vi "wait4.vi"(8 "error In":errorcluster, 9 "JSON string":string, 10 "Step order":string, 11 "process_ID":string) -> (0 "error IO":errorcluster)   [LabVIEW 2020]
uses:
  status/status of power_supply4.vi
  status/emergency stop.vi
  status/pause4.vi
  status/time4.vi
panel:
  out "current time":timestamp
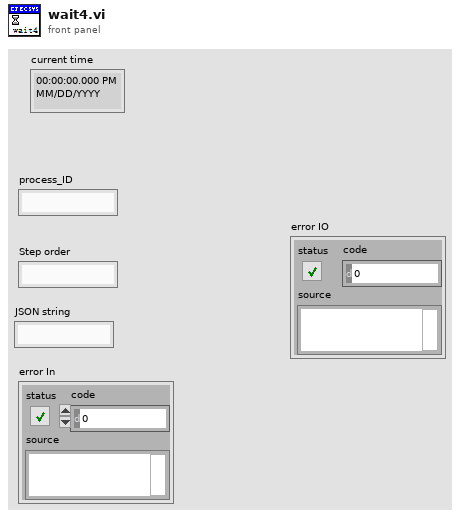
[diagram p1: front panel]
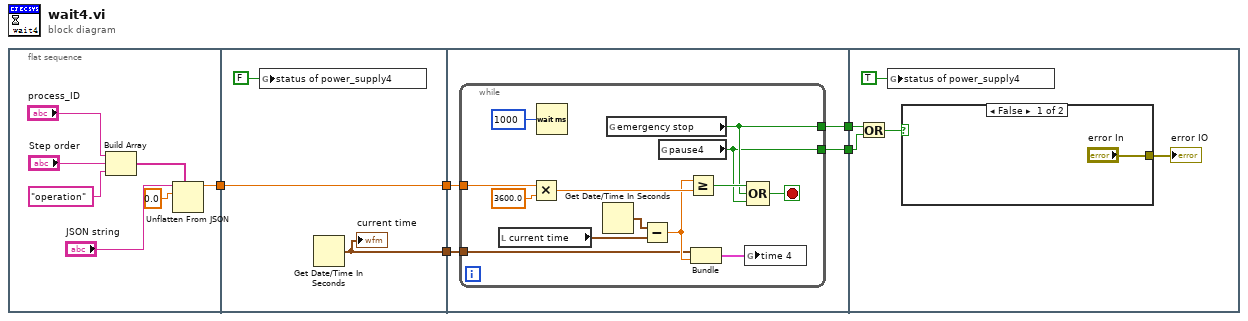
[diagram p0: block diagram]
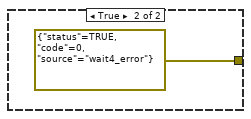
[diagram p2: hidden frame]
diagram:
  n1 = flat-sequence {
    tunnel: [w6] -> w5
    tunnel: w5 -> [w15]
    tunnel: [w15] -> w4
    tunnel: [w13] -> w1
    tunnel: w4 -> [w19]
    tunnel: [w18] -> w3
    tunnel: [w17] -> w2
    tunnel: w1 -> [w16]
    tunnel: w3 -> [w35]
    tunnel: w2 -> [w34]
    frame #0 {
      n2 = Build Array("process_ID", "Step order", "operation" ("string")) -> (w12:string[])
      n3 = Unflatten From JSON(path=w12, JSON string="JSON string", type and defaults=sgl 0.0 ("distance")) -> (value=w6:sgl)  [unwired: 4 in, 1 out]
    }
    frame #1 {
      n4 = global write "status of power_supply4.vi" "status of power_supply4"(FALSE ("status of power_supply4")) -> ()
      n5 = Get Date/Time In Seconds() -> (seconds since 1Jan1904=w13:timestamp)
      "current time" <- w13
    }
    frame #2 {
      n6 = while {
        tunnel: w19 -> [w28]
        tunnel: [w29] -> w18
        tunnel: [w26] -> w17
        tunnel: w16 -> [w20]
        stop <- w31 stop-if-true
        n7 = local read "current time"() -> (w24:timestamp)
        n8 = Multiply(x=w28, y=sgl 3600.0) -> (x*y=w23:sgl)
        n9 = Wait (ms)(milliseconds to wait=u32 1000) -> ()  [unwired: 1 out]
        n10 = Get Date/Time In Seconds() -> (seconds since 1Jan1904=w25:timestamp)
        n11 = global read "emergency stop.vi" "emergency stop"() -> (w29:bool)
        n12 = Subtract(x=w25, y=w24) -> (x-y=w21:dbl)
        n13 = global read "pause4.vi" "pause4"() -> (w26:bool)
        n14 = Greater Or Equal?(x=w21, y=w23) -> (x >= y?=w30:bool)
        n15 = Bundle("seconds since 1Jan1904"=w20, w21) -> (w22:cluster{"seconds since 1Jan1904":timestamp, dbl})  [unwired: 1 in]
        n16 = global write "time4.vi" "time 4"(w22) -> ()
        n17 = Compound Arithmetic op=OR(w30, w29, w26) -> (w31:bool)
      }
    }
    frame #3 {
      n18 = Or(x=w35, y=w34) -> (x .or. y?=w36:bool)
      n19 = global write "status of power_supply4.vi" "status of power_supply4"(TRUE ("status of power_supply4")) -> ()
      n20 = case shown="False" w36 {
        tunnel: ["error In" errorcluster {"status"=TRUE, "code"=0, "source"="wait4_error"} ("error IO")] -> w37
        frame False {
        }
        frame True {
        }
      }
      "error IO" <- w37
    }
  }
